vi "VisualizeStatus.vi"() -> ()   [LabVIEW 2014]
uses:
  VisializeBase_class/VisualizeBase_class.lvclass
  <vilib>/Utility/error.llb/Error Cluster From Error Code.vi
  <vilib>/ErrorRing/Error Ring.xnode
  <userlib>/NIST/NISTErrorLib/NISTErrorLib.lvlib
  <vilib>/event_ctls.llb/usereventprio.ctl
  VisializeBase_class/Requests/clUserEventType.ctl
  Framework/Bus_class/Bus_class.lvlib
  Framework/Bus_class/Broadcast/Typedefs/clDidInit.ctl
  Framework/Bus_class/Bus.lvclass
  <vilib>/Utility/miscctls.llb/LVStringsAndValuesArrayTypeDef_U8.ctl
  Events/EventModule/EventModule.lvlib
  PmuImpairment/PmuImpairModule/PmuImpairModule.lvlib
  NetworkImpairment/NetworkImpairmentModule/NetworkImpairmentModule.lvlib
  FlagImpairment/FlagImpairModule/FlagImpairModule.lvlib
  Events/EventPlugins/EventPluginBaseClass/TypeDefs/clEvtReport.ctl
  Events/EventPlugins/EventPluginBaseClass/EventPluginBaseClass.lvclass
  Events/EventPlugins/EventPluginBaseClass/TypeDefs/clEvtReportArray.ctl
  QMH/Typedefs/clEvtRptArray.ctl
  VisializeBase_class/Typedefs/VisualizeData.ctl
  Events/EventPlugins/EventPluginBaseClass/TypeDefs/dblEvtSignalArray.ctl
  QMH/Typedefs/clEvtRptSignal.ctl
  QMH/Typedefs/clPmuImpairRptArray.ctl
  NetworkImpairment/NetworkImpairmentModule/PublicAPI/Arguments/Broadcasts/dblNetworkTime.ctl
  QMH/Typedefs/clNetImpairmentTime.ctl
  NetworkImpairment/NetworkImpairmentModule/PublicAPI/Arguments/Broadcasts/dblPktLoss.ctl
  QMH/Typedefs/clNetIPktLoss.ctl
  FlagImpairment/FlagImpairModule/PublicAPI/Arguments/Broadcasts/ui32FlagImpairmentArray.ctl
  QMH/Typedefs/clFlagImpairArray.ctl
  VisializeBase_class/Typedefs/clVisualizeData.ctl
panel:
  in  "Scrollbar":i32(c297)=20
  in  "QueName":string="FlagQue"
  out "appended array":errorcluster[][](array[cluster])
  in  "btnStop":bool
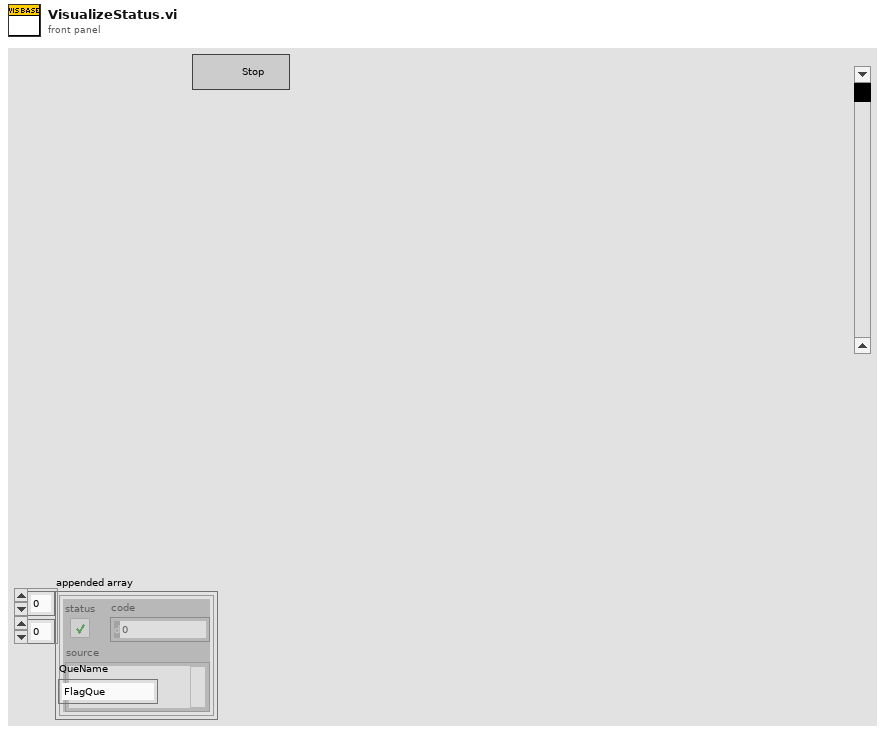
[diagram p1: front panel]
types:
  T1 = typedef "Visualization.lvlib/VisualizeBase_class.lvclass/VisualizeData.ctl" = T2[]
  T2 = typedef "clVisualizeData.ctl" = cluster{"clEvtReportArray":T3, "dblEventSignalArray":T5, "clPmuImpairRptArray":T3, "dblNetworkTime":T6, "dblPktLoss":T7, "FlagImpairArray":T8, "TimeArray":dbl[]}
  T3 = typedef "EventPlugins.lvlib/EventPluginBaseClass.lvclass/clEvtReportArray.ctl" = T4[]
  T4 = typedef "EventPlugins.lvlib/EventPluginBaseClass.lvclass/clEvtReport.ctl" = cluster{"Timestamp":dbl, "Synx":cdb[], "Freq":dbl, "ROCOF":dbl, "ID":i16}
  T5 = typedef "EventPlugins.lvlib/EventPluginBaseClass.lvclass/dblEvtSignalArray.ctl" = dbl[][]
  T6 = typedef "NetworkImpairmentModule.lvlib/dblNetworkTime.ctl" = dbl[]
  T7 = typedef "NetworkImpairmentModule.lvlib/dblPktLoss.ctl" = dbl[]
  T8 = typedef "FlagImpairModule.lvlib/ui32FlagImpairmentArray.ctl" = u32[]
  T9 = typedef "Visualization.lvlib/VisualizeBase_class.lvclass/clRequestEvents.ctl" = cluster{"StopRequest":refnum<user-event>}
  T10 = typedef "Bus_class.lvlib/clBroadcastEvents.ctl" = cluster{"DidInit":refnum<user-event>, "DidStop":refnum<user-event>}
  T11 = typedef "EventModule.lvlib/clBroadcastEvents.ctl" = cluster{"DidInit":refnum<user-event>, "StatusUpdate":refnum<user-event>, "ErrorReport":refnum<user-event>, "DidStop":refnum<user-event>, "ReadEvtConfig":refnum<user-event>, "ReadTimeArray":refnum<user-event>, "ReadEvtParams":refnum<user-event>, "GetEvtReportArray":refnum<user-event>, "ReadPathToPlugin":refnum<user-event>, "GetEvtSignal":refnum<user-event>, "ReadBusNumber":refnum<user-event>}
  T12 = typedef "PmuImpairModule.lvlib/clBroadcastEvents.ctl" = cluster{"DidInit":refnum<user-event>, "StatusUpdate":refnum<user-event>, "ErrorReport":refnum<user-event>, "DidStop":refnum<user-event>, "ImpairConfig":refnum<user-event>, "ImpairParams":refnum<user-event>, "ImpairReports":refnum<user-event>, "PathToPlugin":refnum<user-event>, "BusNumber":refnum<user-event>}
  T13 = typedef "NetworkImpairmentModule.lvlib/clBroadcastEvents.ctl" = cluster{"DidInit":refnum<user-event>, "StatusUpdate":refnum<user-event>, "ErrorReport":refnum<user-event>, "DidStop":refnum<user-event>, "ReadNetImpParams":refnum<user-event>, "ReadLossThreshold":refnum<user-event>, "GetNetworkTime":refnum<user-event>, "GetPktLoss":refnum<user-event>, "ReadPathToPlugin":refnum<user-event>}
  T14 = typedef "FlagImpairModule.lvlib/clBroadcastEvents.ctl" = cluster{"DidInit":refnum<user-event>, "StatusUpdate":refnum<user-event>, "ErrorReport":refnum<user-event>, "DidStop":refnum<user-event>, "ReadFlagImpairConfig":refnum<user-event>, "ReadPluginINIFilePath":refnum<user-event>, "ReadFlagImpairParams":refnum<user-event>, "ReadTimeArray":refnum<user-event>, "GetFlagImpairment":refnum<user-event>}
  T15 = typedef "LVStringsAndValuesArrayTypeDef_U8.ctl" = cluster{"String":string, "Value":u8}[]
  T16 = typedef "Visualization.lvlib/VisualizeBase_class.lvclass/clEvtRptArray.ctl" = cluster{"BusIndex":i32, "clImpairReportArray":T3}
  T17 = typedef "Visualization.lvlib/VisualizeBase_class.lvclass/clPmuImpairRptArray.ctl" = cluster{"BusIndex":i32, "clImpairReportArray":T3}
  T18 = typedef "Visualization.lvlib/VisualizeBase_class.lvclass/clNetImpairmentTime.ctl" = cluster{"BusIndex":i32, "clNetImpairTimeArray":T6}
  T19 = typedef "Visualization.lvlib/VisualizeBase_class.lvclass/clNetIPktLoss.ctl" = cluster{"BusIndex":i32, "clNetPktLoss":T7}
  T20 = typedef "Visualization.lvlib/VisualizeBase_class.lvclass/clFlagImpairArray.ctl" = cluster{"BusIndex":i32, "FlagImpairArray":T8}
  T21 = typedef "Visualization.lvlib/VisualizeBase_class.lvclass/clEvtRptSignal.ctl" = cluster{"BusIndex":i32, "dblEventSignalArray":T5}
  T22 = typedef "Visualization.lvlib/VisualizeBase_class.lvclass/clUserEventType.ctl" = cluster{"BusIndex":i8, "Data":variant}
  T23 = typedef "usereventprio.ctl" = enum32{"high priority", "normal priority"}
  T24 = typedef "Bus_class.lvlib/clDidInit.ctl" = cluster{"Bus":refnum<vi>, "Init?":bool}
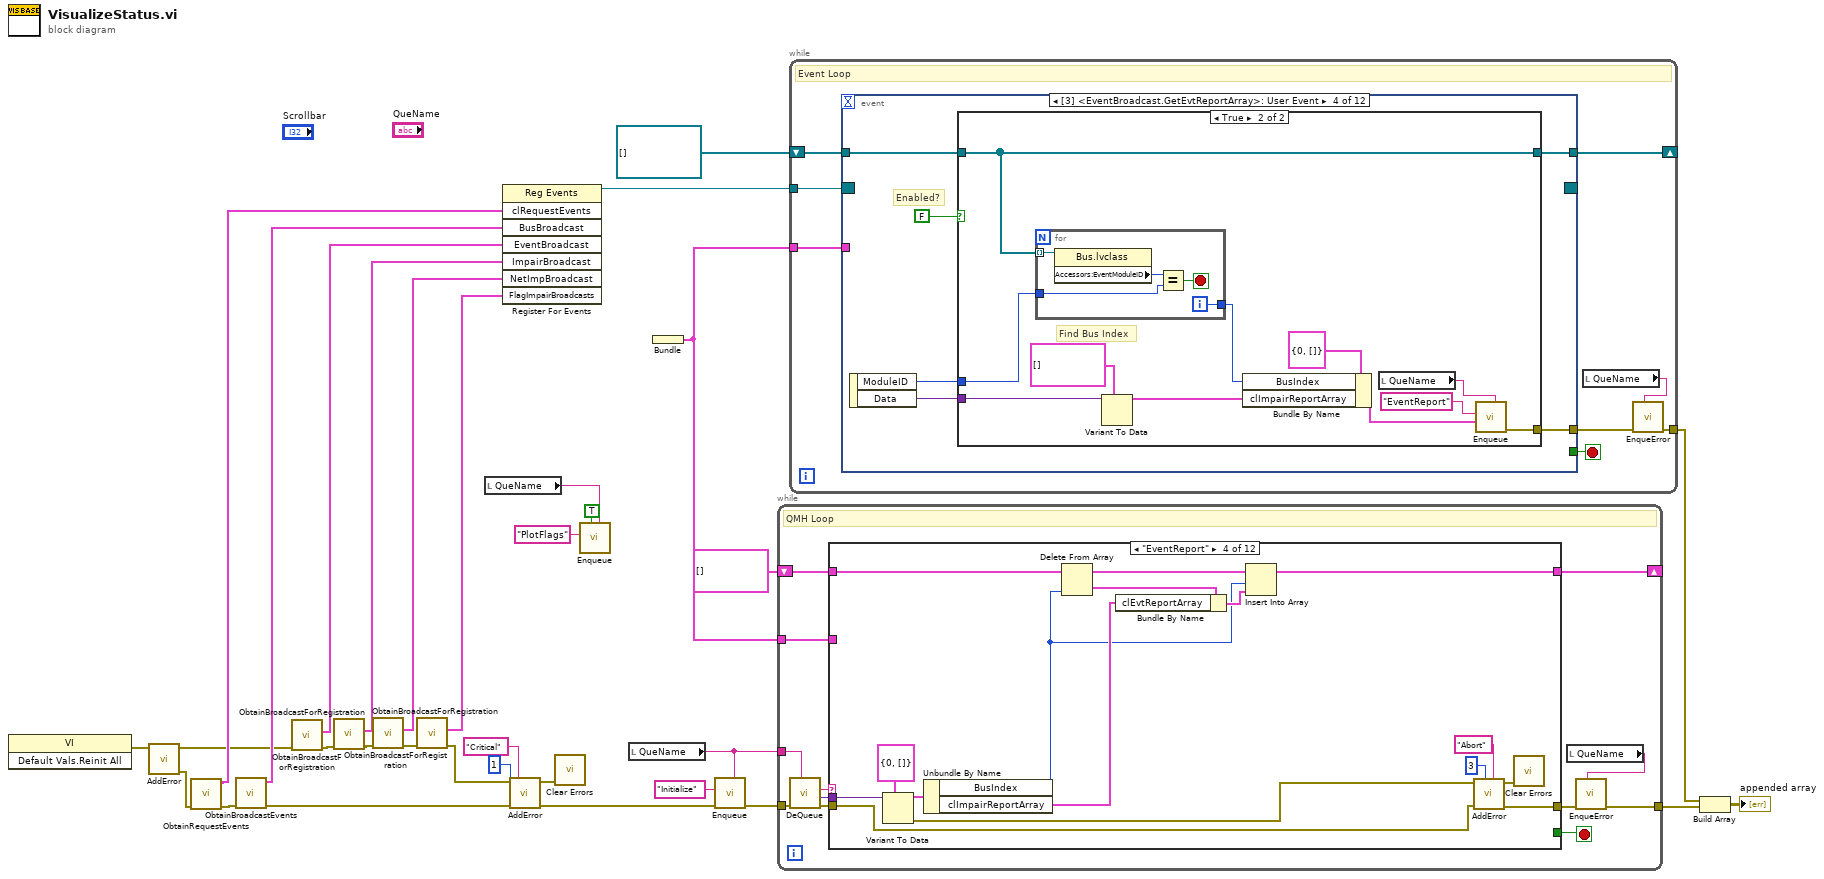
[diagram p0: block diagram]
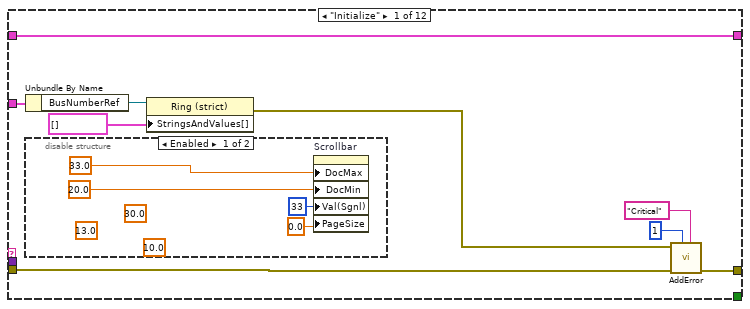
[diagram p2: hidden frame]
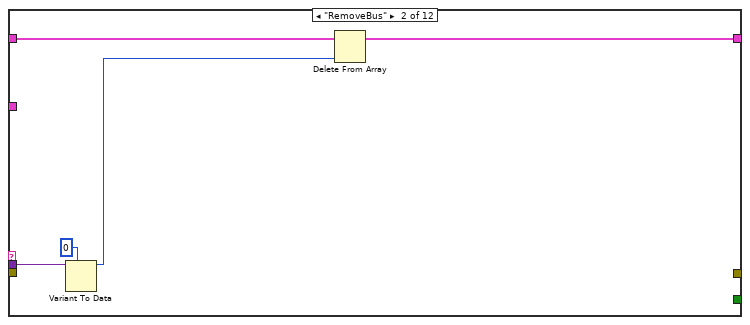
[diagram p4: hidden frame]
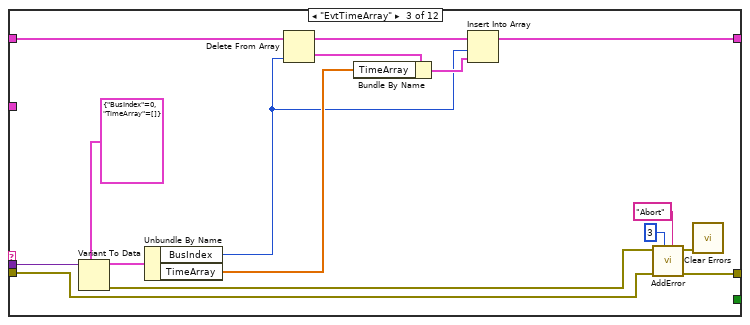
[diagram p5: hidden frame]
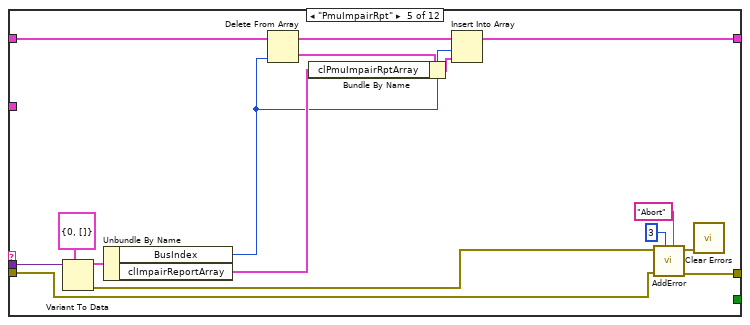
[diagram p6: hidden frame]
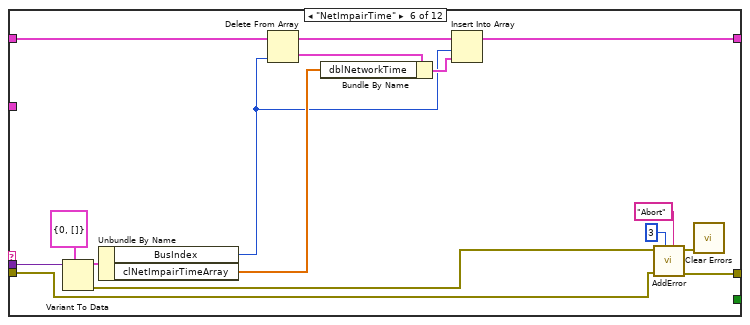
[diagram p7: hidden frame]
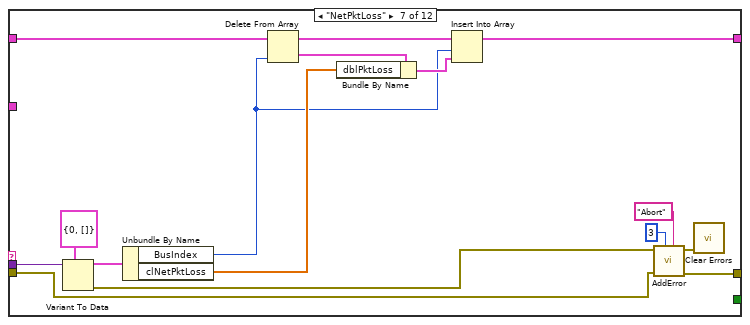
[diagram p8: hidden frame]
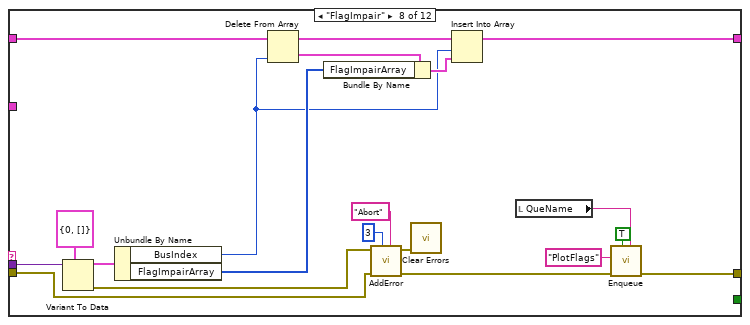
[diagram p9: hidden frame]
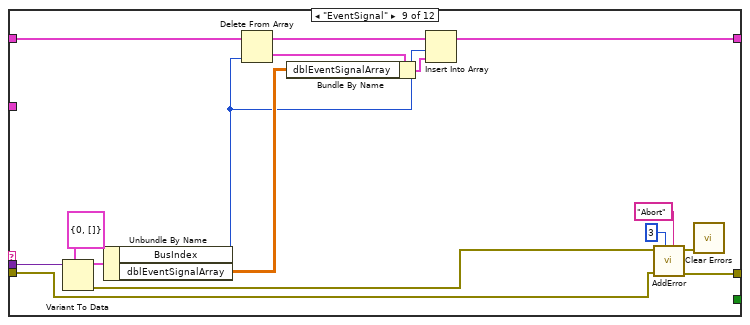
[diagram p10: hidden frame]
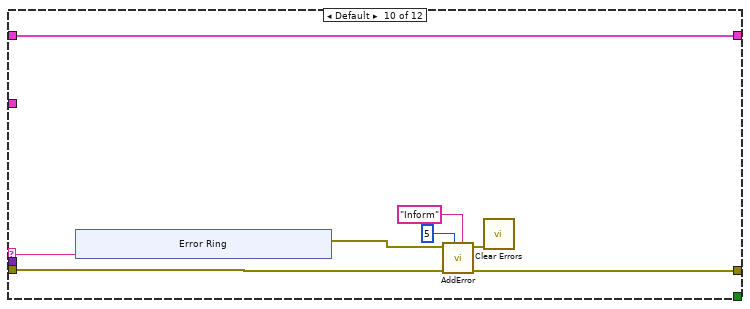
[diagram p11: hidden frame]
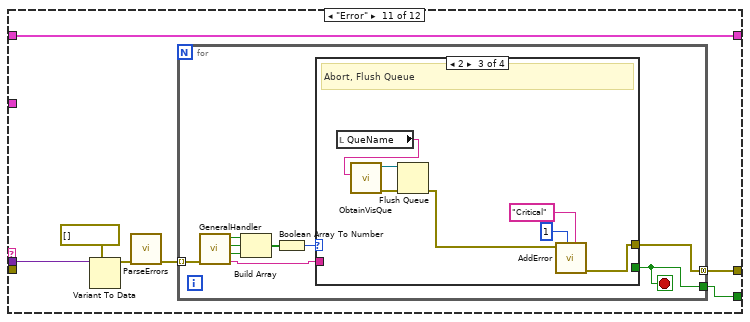
[diagram p12: hidden frame]
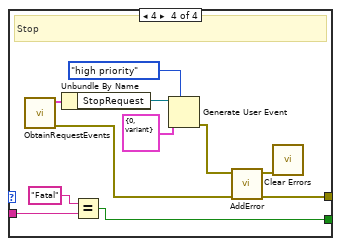
[diagram p15: hidden frame]
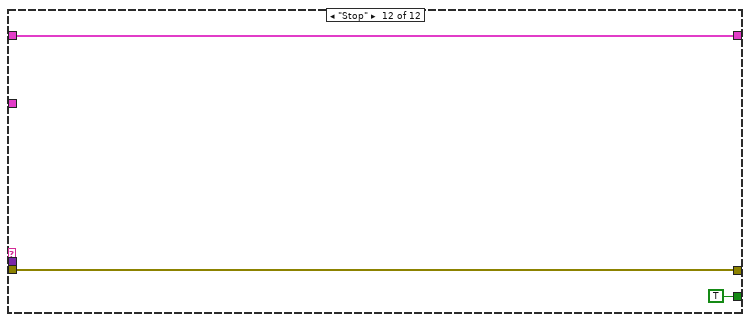
[diagram p16: hidden frame]
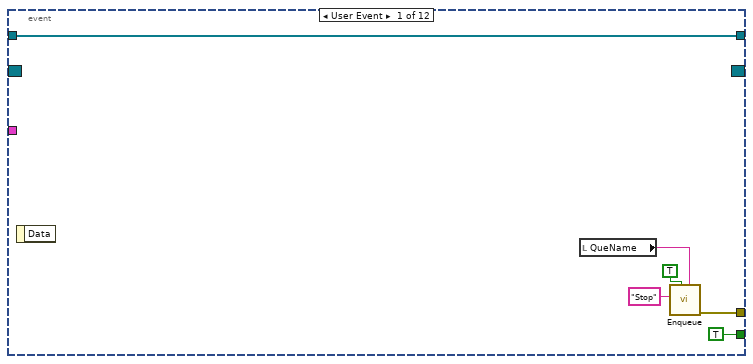
[diagram p17: hidden frame]
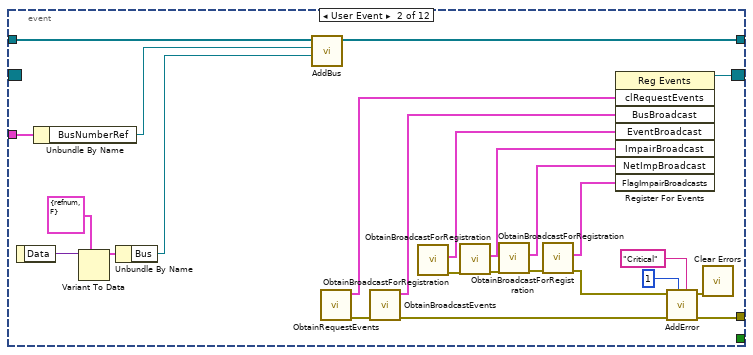
[diagram p18: hidden frame]
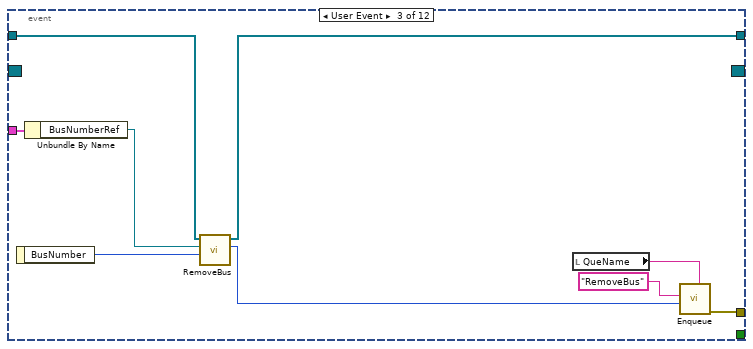
[diagram p19: hidden frame]
diagram:
  n1 = invoke class="VI" method="Default Vals.Reinit All"() -> (error out=w22:errorcluster)  [unwired: 3 in, 2 out]
  n2 = call <userlib>:"AddError.vi"("error in (no error)"=w22) -> ("ErrorArray"=w21:errorcluster[], "error out"=w13:errorcluster)  [unwired: 9 in]
  n3 = call "ObtainRequestEvents.vi"("Error"=w21) -> ("Error"=w26:errorcluster[], "clRequestEvents"=w31:T9)  [unwired: 9 in]
  n4 = call "ObtainBroadcastEvents.vi"("ErrorArray"=w26) -> ("ErrorArray"=w12:errorcluster[], "BusBroadcast"=w25:T10)  [unwired: 9 in]
  n5 = call "ObtainBroadcastForRegistration.vi"("error in (no error)"=w13) -> ("error out"=w16:errorcluster, "EventBroadcast"=w20:T11)  [unwired: 9 in]
  n6 = call "ObtainBroadcastForRegistration.vi"("error in (no error)"=w16) -> ("error out"=w15:errorcluster, "ImpairBroadcast"=w19:T12)  [unwired: 9 in]
  n7 = call "ObtainBroadcastForRegistration.vi"("error in (no error)"=w15) -> ("error out"=w14:errorcluster, "NetImpBroadcast"=w18:T13)  [unwired: 9 in]
  n8 = call "ObtainBroadcastForRegistration.vi"("error in (no error)"=w14) -> ("error out"=w11:errorcluster, "FlagImpairBroadcasts"=w17:T14)  [unwired: 9 in]
  n9 = local read "QueName"() -> (w3:string)
  n10 = register-events(w31, w25, w20, w19, w18, w17) -> (reference out=w30:refnum<event-registration>)  [unwired: 2 in, 1 out]
  n11 = call <userlib>:"AddError.vi"("Severity"="Critical" ("String"), "Priority"=u8 1, "ErrorArray"=w12, "error in (no error)"=w11) -> ("ErrorArray"=w8:errorcluster[], "error out"=w5:errorcluster)  [unwired: 6 in]
  n12 = call <vilib>:"Clear Errors.vi"("error in (no error)"=w5) -> ()  [unwired: 5 in, 2 out]
  n13 = call "Enqueue.vi"("QueName"=w3, "Priority? (F)"=TRUE, "Message"="PlotFlags") -> ()  [unwired: 8 in, 1 out]
  n14 = local read "QueName"() -> (w4:string)
  n15 = Bundle() -> (w6:cluster{void}, w24)  [unwired: 1 in]
  n16 = call "Enqueue.vi"("QueName"=w4, "Error"=w8, "Message"="Initialize") -> ("Error"=w32:errorcluster[])  [unwired: 8 in]
  n17 = while {
    tunnel: w32 -> [w45]
    tunnel: [w39] -> w29
    tunnel: w6 -> [w38]
    shift-right: [w36] -> _
    shift-left: T1 [] ("VisualizeData") -> [w37]
    tunnel: w4 -> [w35]
    stop <- w40 stop-if-true
    # "QMH Loop"
    n18 = call "DeQueue.vi"("QueName"=w35, "Error"=w45) -> ("Error"=w42:errorcluster[], "Data"=w43:variant, "Message"=w44:string)  [unwired: 7 in]
    n19 = case shown="\"EventReport\"" w44 {
      selector: w44 -> [_ _ _ _ _ _ _ _ _ w190 _ _]
      tunnel: w43 -> [_ w66 w69 w98 w114 w130 w146 w166 w182 _ w204 _]
      tunnel: w42 -> [w51 _ w68 w83 w99 w115 w131 w152 w167 w188 _ w233]
      tunnel: [w50 _ w67 w88 w104 w120 w136 w150 w172 w187 w200 w233] -> w41
      tunnel: [_ _ _ _ _ _ _ _ _ _ w199 TRUE] -> w40
      tunnel: w38 -> [w54 _ _ _ _ _ _ _ _ _ _ _]
      tunnel: w37 -> [w46 w64 w71 w94 w110 w126 w142 w162 w178 w183 w198 w232]
      tunnel: [w46 w63 w70 w95 w111 w127 w143 w163 w179 w183 w198 w232] -> w36
      frame "Initialize" {
        n20 = Unbundle By Name(w54) -> ("BusNumberRef"=w53:refnum<vi>)
        n21 = disable-structure shown="Enabled" {
          frame Enabled {
            w55 = 10.0 ("Y Scale.Range:Increment")
            w59 = 30.0 ("Y Scale.Range:Maximum")
            w58 = 13.0 ("Y Scale.Range:Maximum")
            n22 = property on="Scrollbar" class="Scroll (strict)"("DocMax"=33.0 ("Doc Max"), "DocMin"=20.0 ("Doc Min"), "Val(Sgnl)"=33 ("Scrollbar"), "PageSize"=0.0 ("Page Size")) -> ()  [unwired: 2 in, 2 out]
          }
          frame Disabled {
          }
        }
        n23 = property class="Ring (strict)"(reference=w53, "StringsAndValues[]"=T15 [] ("Strings And Values []")) -> (error out=w49:errorcluster)  [unwired: 1 in, 1 out]
        n24 = call <userlib>:"AddError.vi"("Severity"="Critical" ("String"), "Priority"=u8 1, "ErrorArray"=w51, "error in (no error)"=w49) -> ("ErrorArray"=w50:errorcluster[])  [unwired: 6 in, 1 out]
      }
      frame "RemoveBus" {
        n25 = Variant To Data(type=0, Variant=w66) -> (data=w62:i32)  [unwired: 1 in, 1 out]
        n26 = Delete From Array(array=w64, index=w62) -> (array with subset deleted=w63:T1)  [unwired: 1 in, 1 out]
      }
      frame "EvtTimeArray" {
        n27 = Variant To Data(type=cluster{"BusIndex":i32, "TimeArray":dbl[]} {"BusIndex"=0, "TimeArray"=[]} ("cluster"), Variant=w69) -> (data=w78:cluster{"BusIndex":i32, "TimeArray":dbl[]}, error out=w82:errorcluster)  [unwired: 1 in]
        n28 = Unbundle By Name(w78) -> ("BusIndex"=w73:i32, "TimeArray"=w75:dbl[])
        n29 = Delete From Array(array=w71, index=w73) -> (deleted portion=w76:T2, array with subset deleted=w77:T1)  [unwired: 1 in]
        n30 = Bundle By Name(cluster=w76, "TimeArray"=w75) -> (w74:T2)
        n31 = Insert Into Array(array=w77, index=w73, new element=w74) -> (w70:T1)
        n32 = call <userlib>:"AddError.vi"("Severity"="Abort" ("String"), "Priority"=u8 3, "ErrorArray"=w68, "error in (no error)"=w82) -> ("ErrorArray"=w67:errorcluster[], "error out"=w81:errorcluster)  [unwired: 6 in]
        n33 = call <vilib>:"Clear Errors.vi"("error in (no error)"=w81) -> ()  [unwired: 5 in, 2 out]
      }
      frame "EventReport" {
        n34 = Variant To Data(type=T16 {"BusIndex"=0, "clImpairReportArray"=[]} ("clEvtReportArray"), Variant=w98) -> (data=w96:T16, error out=w87:errorcluster)  [unwired: 1 in]
        n35 = Unbundle By Name(w96) -> ("BusIndex"=w89:i32, "clImpairReportArray"=w91:T3)
        n36 = Delete From Array(array=w94, index=w89) -> (deleted portion=w92:T2, array with subset deleted=w93:T1)  [unwired: 1 in]
        n37 = Bundle By Name(cluster=w92, "clEvtReportArray"=w91) -> (w90:T2)
        n38 = Insert Into Array(array=w93, index=w89, new element=w90) -> (w95:T1)
        n39 = call <userlib>:"AddError.vi"("Severity"="Abort" ("String"), "Priority"=u8 3, "ErrorArray"=w83, "error in (no error)"=w87) -> ("ErrorArray"=w88:errorcluster[], "error out"=w86:errorcluster)  [unwired: 6 in]
        n40 = call <vilib>:"Clear Errors.vi"("error in (no error)"=w86) -> ()  [unwired: 5 in, 2 out]
      }
      frame "PmuImpairRpt" {
        n41 = Variant To Data(type=T17 {"BusIndex"=0, "clImpairReportArray"=[]} ("clImpairReportArray"), Variant=w114) -> (data=w112:T17, error out=w103:errorcluster)  [unwired: 1 in]
        n42 = Unbundle By Name(w112) -> ("BusIndex"=w105:i32, "clImpairReportArray"=w107:T3)
        n43 = Delete From Array(array=w110, index=w105) -> (deleted portion=w108:T2, array with subset deleted=w109:T1)  [unwired: 1 in]
        n44 = Bundle By Name(cluster=w108, "clPmuImpairRptArray"=w107) -> (w106:T2)
        n45 = Insert Into Array(array=w109, index=w105, new element=w106) -> (w111:T1)
        n46 = call <userlib>:"AddError.vi"("Severity"="Abort" ("String"), "Priority"=u8 3, "ErrorArray"=w99, "error in (no error)"=w103) -> ("ErrorArray"=w104:errorcluster[], "error out"=w102:errorcluster)  [unwired: 6 in]
        n47 = call <vilib>:"Clear Errors.vi"("error in (no error)"=w102) -> ()  [unwired: 5 in, 2 out]
      }
      frame "NetImpairTime" {
        n48 = Variant To Data(type=T18 {"BusIndex"=0, "clNetImpairTimeArray"=[]} ("clImpairReportArray"), Variant=w130) -> (data=w128:T18, error out=w119:errorcluster)  [unwired: 1 in]
        n49 = Unbundle By Name(w128) -> ("BusIndex"=w121:i32, "clNetImpairTimeArray"=w123:T6)
        n50 = Delete From Array(array=w126, index=w121) -> (deleted portion=w124:T2, array with subset deleted=w125:T1)  [unwired: 1 in]
        n51 = Bundle By Name(cluster=w124, "dblNetworkTime"=w123) -> (w122:T2)
        n52 = Insert Into Array(array=w125, index=w121, new element=w122) -> (w127:T1)
        n53 = call <userlib>:"AddError.vi"("Severity"="Abort" ("String"), "Priority"=u8 3, "ErrorArray"=w115, "error in (no error)"=w119) -> ("ErrorArray"=w120:errorcluster[], "error out"=w118:errorcluster)  [unwired: 6 in]
        n54 = call <vilib>:"Clear Errors.vi"("error in (no error)"=w118) -> ()  [unwired: 5 in, 2 out]
      }
      frame "NetPktLoss" {
        n55 = Variant To Data(type=T19 {"BusIndex"=0, "clNetPktLoss"=[]} ("clNetPktLoss"), Variant=w146) -> (data=w144:T19, error out=w135:errorcluster)  [unwired: 1 in]
        n56 = Unbundle By Name(w144) -> ("BusIndex"=w137:i32, "clNetPktLoss"=w139:T7)
        n57 = Delete From Array(array=w142, index=w137) -> (deleted portion=w140:T2, array with subset deleted=w141:T1)  [unwired: 1 in]
        n58 = Bundle By Name(cluster=w140, "dblPktLoss"=w139) -> (w138:T2)
        n59 = Insert Into Array(array=w141, index=w137, new element=w138) -> (w143:T1)
        n60 = call <userlib>:"AddError.vi"("Severity"="Abort" ("String"), "Priority"=u8 3, "ErrorArray"=w131, "error in (no error)"=w135) -> ("ErrorArray"=w136:errorcluster[], "error out"=w134:errorcluster)  [unwired: 6 in]
        n61 = call <vilib>:"Clear Errors.vi"("error in (no error)"=w134) -> ()  [unwired: 5 in, 2 out]
      }
      frame "FlagImpair" {
        n62 = Variant To Data(type=T20 {"BusIndex"=0, "FlagImpairArray"=[]} ("clFlagImpairArray"), Variant=w166) -> (data=w164:T20, error out=w156:errorcluster)  [unwired: 1 in]
        n63 = Unbundle By Name(w164) -> ("BusIndex"=w157:i32, "FlagImpairArray"=w159:T8)
        n64 = Delete From Array(array=w162, index=w157) -> (deleted portion=w160:T2, array with subset deleted=w161:T1)  [unwired: 1 in]
        n65 = Bundle By Name(cluster=w160, "FlagImpairArray"=w159) -> (w158:T2)
        n66 = call <userlib>:"AddError.vi"("Severity"="Abort" ("String"), "Priority"=u8 3, "ErrorArray"=w152, "error in (no error)"=w156) -> ("ErrorArray"=w151:errorcluster[], "error out"=w155:errorcluster)  [unwired: 6 in]
        n67 = call <vilib>:"Clear Errors.vi"("error in (no error)"=w155) -> ()  [unwired: 5 in, 2 out]
        n68 = Insert Into Array(array=w161, index=w157, new element=w158) -> (w163:T1)
        n69 = local read "QueName"() -> (w147:string)
        n70 = call "Enqueue.vi"("QueName"=w147, "Priority? (F)"=TRUE, "Error"=w151, "Message"="PlotFlags") -> ("Error"=w150:errorcluster[])  [unwired: 7 in]
      }
      frame "EventSignal" {
        n71 = Variant To Data(type=T21 {"BusIndex"=0, "dblEventSignalArray"=[]} ("clEvtReportArray"), Variant=w182) -> (data=w180:T21, error out=w171:errorcluster)  [unwired: 1 in]
        n72 = Unbundle By Name(w180) -> ("BusIndex"=w173:i32, "dblEventSignalArray"=w175:T5)
        n73 = Delete From Array(array=w178, index=w173) -> (deleted portion=w176:T2, array with subset deleted=w177:T1)  [unwired: 1 in]
        n74 = Bundle By Name(cluster=w176, "dblEventSignalArray"=w175) -> (w174:T2)
        n75 = Insert Into Array(array=w177, index=w173, new element=w174) -> (w179:T1)
        n76 = call <userlib>:"AddError.vi"("Severity"="Abort" ("String"), "Priority"=u8 3, "ErrorArray"=w167, "error in (no error)"=w171) -> ("ErrorArray"=w172:errorcluster[], "error out"=w170:errorcluster)  [unwired: 6 in]
        n77 = call <vilib>:"Clear Errors.vi"("error in (no error)"=w170) -> ()  [unwired: 5 in, 2 out]
      }
      frame Default {
        n78 = xnode "Error Ring"("parameter 0"=w190) -> ("error out"=w189:errorcluster)
        n79 = call <userlib>:"AddError.vi"("Severity"="Inform" ("String"), "Priority"=u8 5, "ErrorArray"=w188, "error in (no error)"=w189) -> ("ErrorArray"=w187:errorcluster[], "error out"=w186:errorcluster)  [unwired: 6 in]
        n80 = call <vilib>:"Clear Errors.vi"("error in (no error)"=w186) -> ()  [unwired: 5 in, 2 out]
      }
      frame "Error" {
        n81 = Variant To Data(type=errorcluster[] [], Variant=w204) -> (data=w202:errorcluster[])  [unwired: 1 in, 1 out]
        n82 = call <userlib>:"ParseErrors.vi"("ErrorArray"=w202) -> ("ErrorArray"=w201:errorcluster[])  [unwired: 8 in, 2 out]
        n83 = for {
          tunnel: w201 -> [w213] mode=indexing
          tunnel: [w207] -> w200 mode=concatenating
          tunnel: [w205] -> w199
          stop <- w205 stop-if-true
          n84 = call <userlib>:"GeneralHandler.vi"("error in (no error)"=w213) -> ("Severity"=w206:string, "Stop"=w210:bool, "Abort"=w211:bool, "Continue"=w212:bool)  [unwired: 7 in]
          n85 = Build Array(w212, w211, w210) -> (w209:bool[])
          n86 = Boolean Array To Number(Boolean array=w209) -> (number=w208:u32)
          n87 = case shown="2" w208 {
            tunnel: [_ _ w218 w229] -> w207
            tunnel: w206 -> [_ _ _ w223]
            tunnel: [_ _ _ w221] -> w205
            frame 0, Default {
              # "No Dialog"
            }
            frame 1 {
              # "Continue"
            }
            frame 2 {
              # "Abort, Flush Queue"
              n88 = local read "QueName"() -> (w214:string)
              n89 = call "ObtainVisQue.vi"("QueName"=w214) -> ("error out"=w220:errorcluster, "queue out"=w219:refnum<queue>)  [unwired: 9 in]
              n90 = Flush Queue(queue=w219, error in (no error)=w220) -> (error out=w217:errorcluster)  [unwired: 2 out]
              n91 = call <userlib>:"AddError.vi"("Severity"="Critical" ("String"), "Priority"=u8 1, "error in (no error)"=w217) -> ("ErrorArray"=w218:errorcluster[])  [unwired: 7 in, 1 out]
            }
            frame 4 {
              # "Stop"
              n92 = call "ObtainRequestEvents.vi"() -> ("Error"=w227:errorcluster[], "clRequestEvents"=w231:T9)  [unwired: 10 in]
              n93 = Unbundle By Name(w231) -> ("StopRequest"=w230:refnum<user-event>)
              n94 = Equal?(x="Fatal", y=w223) -> (x = y?=w221:bool)
              n95 = Generate User Event(priority (normal)=usereventprio."high priority", user event=w230, event data cluster=T22 {"BusIndex"=0, "Data"=variant} ("event data")) -> (error out=w228:errorcluster)  [unwired: 1 in, 1 out]
              n96 = call <userlib>:"AddError.vi"("ErrorArray"=w227, "error in (no error)"=w228) -> ("ErrorArray"=w229:errorcluster[], "error out"=w224:errorcluster)  [unwired: 8 in]
              n97 = call <vilib>:"Clear Errors.vi"("error in (no error)"=w224) -> ()  [unwired: 5 in, 2 out]
            }
          }
        }
      }
      frame "Stop" {
      }
    }
    n98 = local read "QueName"() -> (w34:string)
    n99 = call "EnqueError.vi"("QueName"=w34, "Error"=w41) -> ("Error"=w39:errorcluster[])  [unwired: 9 in]
  }
  n100 = while {
    tunnel: w30 -> [w242]
    tunnel: [w239] -> w28
    tunnel: w6 -> [w238]
    shift-right: [w236] -> _
    shift-left: refnum<class "Bus.lvclass">[] [] -> [w237]
    stop <- w241 stop-if-true
    # "Event Loop"
    n101 = event shown="[3] <EventBroadcast.GetEvtReportArray>: User Event" {
      selector: w242 -> [_ _ _ _ _ _ _ _ _ _ _ _]
      dyn-events: [_ w257 _ _ _ _ _ _ _ _ _ _] -> _
      timeout: _ -> [_ _ _ _ _ _ _ _ _ _ _ _]
      tunnel: [TRUE _ _ _ _ _ _ _ _ _ _ _] -> w241
      tunnel: [w247 w260 w278 w285 w311 w336 w359 w382 w405 w428 _ w461] -> w240
      tunnel: w238 -> [_ w270 w282 _ _ _ _ _ _ _ _ _]
      tunnel: w237 -> [w244 w269 w281 w288 w309 w339 w362 w385 w408 w431 w449 w455]
      tunnel: [w244 w266 w280 w283 w310 w334 w357 w380 w403 w426 w449 w455] -> w236
      event User Event {
        n102 = event-data() -> ()  [unwired: 1 in, 1 out]
        n103 = local read "QueName"() -> (w243:string)
        n104 = call "Enqueue.vi"("QueName"=w243, "Priority? (F)"=TRUE, "Message"="Stop") -> ("Error"=w247:errorcluster[])  [unwired: 8 in]
      }
      event User Event {
        n105 = event-data() -> ("Data"=w273:variant)  [unwired: 1 in]
        n106 = Unbundle By Name(w270) -> ("BusNumberRef"=w268:refnum<vi>)
        n107 = Variant To Data(type=T24 {"Bus"=refnum, "Init?"=FALSE} ("clBusDidInit"), Variant=w273) -> (data=w271:T24)  [unwired: 1 in, 1 out]
        n108 = Unbundle By Name(w271) -> ("Bus"=w267:refnum<vi>)
        n109 = call "AddBus.vi"("BusRef"=w267, "BusNumberRef"=w268, "BusArray"=w269) -> ("BusArray"=w266:refnum<class "Bus.lvclass">[])  [unwired: 8 in]
        n110 = call "ObtainRequestEvents.vi"() -> ("Error"=w252:errorcluster[], "clRequestEvents"=w250:T9)  [unwired: 10 in]
        n111 = call "ObtainBroadcastEvents.vi"("ErrorArray"=w252) -> ("ErrorArray"=w251:errorcluster[], "BusBroadcast"=w249:T10)  [unwired: 9 in]
        n112 = call "ObtainBroadcastForRegistration.vi"() -> ("error out"=w265:errorcluster, "EventBroadcast"=w256:T11)  [unwired: 10 in]
        n113 = call "ObtainBroadcastForRegistration.vi"("error in (no error)"=w265) -> ("error out"=w264:errorcluster, "ImpairBroadcast"=w255:T12)  [unwired: 9 in]
        n114 = call "ObtainBroadcastForRegistration.vi"("error in (no error)"=w264) -> ("error out"=w263:errorcluster, "NetImpBroadcast"=w254:T13)  [unwired: 9 in]
        n115 = call "ObtainBroadcastForRegistration.vi"("error in (no error)"=w263) -> ("error out"=w258:errorcluster, "FlagImpairBroadcasts"=w253:T14)  [unwired: 9 in]
        n116 = register-events(w250, w249, w256, w255, w254, w253) -> (reference out=w257:refnum<event-registration>)  [unwired: 2 in, 1 out]
        n117 = call <userlib>:"AddError.vi"("Severity"="Critical" ("String"), "Priority"=u8 1, "ErrorArray"=w251, "error in (no error)"=w258) -> ("ErrorArray"=w260:errorcluster[], "error out"=w259:errorcluster)  [unwired: 6 in]
        n118 = call <vilib>:"Clear Errors.vi"("error in (no error)"=w259) -> ()  [unwired: 5 in, 2 out]
      }
      event User Event {
        n119 = event-data() -> ("BusNumber"=w275:i8)  [unwired: 1 in]
        n120 = Unbundle By Name(w282) -> ("BusNumberRef"=w279:refnum<vi>)
        n121 = call "RemoveBus.vi"("BusArray"=w281, "BusNumberRef"=w279, "BusNumber"=w275) -> ("BusArray"=w280:refnum<class "Bus.lvclass">[], "BusIndex"=w277:i32)  [unwired: 6 in]
        n122 = local read "QueName"() -> (w274:string)
        n123 = call "Enqueue.vi"("QueName"=w274, "Data"=w277, "Message"="RemoveBus") -> ("Error"=w278:errorcluster[])  [unwired: 8 in]
      }
      event User Event {
        # "Enabled?"
        n124 = event-data() -> ("ModuleID"=w287:i32, "Data"=w286:variant)  [unwired: 1 in]
        n125 = case shown="True" FALSE {
          tunnel: w288 -> [w289 w291]
          tunnel: w287 -> [_ w300]
          tunnel: w286 -> [_ w298]
          tunnel: [_ w295] -> w285
          tunnel: [w289 w291] -> w283
          frame False {
          }
          frame True {
            # "Find Bus Index"
            n126 = for {
              tunnel: w291 -> [w305] mode=indexing
              tunnel: w300 -> [w303]
              tunnel: [w301] -> w299
              i -> [w301]
              stop <- w302 stop-if-true
              n127 = property class="Bus.lvclass"(reference=w305) -> ("Accessors:EventModuleID"=w304:i32)  [unwired: 1 in, 2 out]
              n128 = Equal?(x=w304, y=w303) -> (x = y?=w302:bool)
            }
            n129 = Variant To Data(type=T3 [] ("clEvtReportArray"), Variant=w298) -> (data=w296:T3)  [unwired: 1 in, 1 out]
            n130 = Bundle By Name(cluster=T16 {"BusIndex"=0, "clImpairReportArray"=[]} ("clEvtReportArray"), "BusIndex"=w299, "clImpairReportArray"=w296) -> (w294:T16)
            n131 = local read "QueName"() -> (w290:string)
            n132 = call "Enqueue.vi"("QueName"=w290, "Data"=w294, "Message"="EventReport") -> ("Error"=w295:errorcluster[])  [unwired: 8 in]
          }
        }
      }
      event User Event {
        w306 = TRUE  # Enabled?
        n133 = event-data() -> ("ModuleID"=w308:i32, "Data"=w307:variant)  [unwired: 1 in]
        n134 = case shown="True" w306 {
          tunnel: [w312 w328] -> w310
          tunnel: w309 -> [w312 w328]
          tunnel: w308 -> [_ w325]
          tunnel: w307 -> [_ w327]
          tunnel: [_ w315] -> w311
          frame False {
          }
          frame True {
            n135 = Variant To Data(type=dbl[] [], Variant=w327) -> (data=w324:dbl[], error out=w320:errorcluster)  [unwired: 1 in]
            n136 = for {
              tunnel: w328 -> [w333] mode=indexing
              tunnel: w325 -> [w331]
              tunnel: [w329] -> w314
              i -> [w329]
              stop <- w330 stop-if-true
              # "Find Bus Index"
              n137 = property class="Bus.lvclass"(reference=w333) -> ("Accessors:EventModuleID"=w332:i32)  [unwired: 1 in, 2 out]
              n138 = Equal?(x=w332, y=w331) -> (x = y?=w330:bool)
            }
            n139 = call <userlib>:"AddError.vi"("Severity"="Critical" ("String"), "Priority"=u8 1, "error in (no error)"=w320) -> ("ErrorArray"=w316:errorcluster[], "error out"=w319:errorcluster)  [unwired: 7 in]
            n140 = call <vilib>:"Clear Errors.vi"("error in (no error)"=w319) -> ()  [unwired: 5 in, 2 out]
            n141 = Bundle(w314, w324) -> (w323:cluster{i32, dbl[]})  [unwired: 1 in]
            n142 = To Variant(anything=w323) -> (Variant=w322:variant)
            n143 = local read "QueName"() -> (w313:string)
            n144 = call "Enqueue.vi"("QueName"=w313, "Error"=w316, "Data"=w322, "Message"="EvtTimeArray") -> ("Error"=w315:errorcluster[])  [unwired: 7 in]
          }
        }
      }
      event User Event {
        # "Enabled?"
        n145 = event-data() -> ("ModuleID"=w338:i32, "Data"=w337:variant)  [unwired: 1 in]
        n146 = case shown="False" FALSE {
          tunnel: w339 -> [w340 w342]
          tunnel: w338 -> [_ w351]
          tunnel: w337 -> [_ w349]
          tunnel: [_ w346] -> w336
          tunnel: [w340 w342] -> w334
          frame False {
          }
          frame True {
            # "Find Bus Index"
            n147 = for {
              tunnel: w342 -> [w356] mode=indexing
              tunnel: w351 -> [w354]
              tunnel: [w352] -> w350
              i -> [w352]
              stop <- w353 stop-if-true
              n148 = property class="Bus.lvclass"(reference=w356) -> ("Accessors:EventModuleID"=w355:i32)  [unwired: 1 in, 2 out]
              n149 = Equal?(x=w355, y=w354) -> (x = y?=w353:bool)
            }
            n150 = Variant To Data(type=T5 [] ("dblEventSignalArray"), Variant=w349) -> (data=w347:T5)  [unwired: 1 in, 1 out]
            n151 = Bundle By Name(cluster=T21 {"BusIndex"=0, "dblEventSignalArray"=[]} ("clEvtReportArray"), "BusIndex"=w350, "dblEventSignalArray"=w347) -> (w345:T21)
            n152 = local read "QueName"() -> (w341:string)
            n153 = call "Enqueue.vi"("QueName"=w341, "Data"=w345, "Message"="EventSignal") -> ("Error"=w346:errorcluster[])  [unwired: 8 in]
          }
        }
      }
      event User Event {
        # "Enabled?"
        n154 = event-data() -> ("ModuleID"=w361:i32, "Data"=w360:variant)  [unwired: 1 in]
        n155 = case shown="True" FALSE {
          tunnel: w362 -> [w363 w365]
          tunnel: w361 -> [_ w374]
          tunnel: w360 -> [_ w372]
          tunnel: [_ w369] -> w359
          tunnel: [w363 w365] -> w357
          frame False {
          }
          frame True {
            # "Find Bus Index"
            n156 = for {
              tunnel: w365 -> [w379] mode=indexing
              tunnel: w374 -> [w377]
              tunnel: [w375] -> w373
              i -> [w375]
              stop <- w376 stop-if-true
              n157 = property class="Bus.lvclass"(reference=w379) -> ("Accessors:EventModuleID"=w378:i32)  [unwired: 1 in, 2 out]
              n158 = Equal?(x=w378, y=w377) -> (x = y?=w376:bool)
            }
            n159 = Variant To Data(type=T3 [] ("clEvtReportArray"), Variant=w372) -> (data=w370:T3)  [unwired: 1 in, 1 out]
            n160 = Bundle By Name(cluster=T17 {"BusIndex"=0, "clImpairReportArray"=[]} ("clEvtReportArray"), "BusIndex"=w373, "clImpairReportArray"=w370) -> (w368:T17)
            n161 = local read "QueName"() -> (w364:string)
            n162 = call "Enqueue.vi"("QueName"=w364, "Data"=w368, "Message"="PmuImpairRpt") -> ("Error"=w369:errorcluster[])  [unwired: 8 in]
          }
        }
      }
      event User Event {
        # "Enabled?"
        n163 = event-data() -> ("ModuleID"=w384:i32, "Data"=w383:variant)  [unwired: 1 in]
        n164 = case shown="False" FALSE {
          tunnel: w385 -> [w386 w388]
          tunnel: w384 -> [_ w397]
          tunnel: w383 -> [_ w395]
          tunnel: [_ w392] -> w382
          tunnel: [w386 w388] -> w380
          frame False {
          }
          frame True {
            # "Find Bus Index"
            n165 = for {
              tunnel: w388 -> [w402] mode=indexing
              tunnel: w397 -> [w400]
              tunnel: [w398] -> w396
              i -> [w398]
              stop <- w399 stop-if-true
              n166 = property class="Bus.lvclass"(reference=w402) -> ("Accessors:EventModuleID"=w401:i32)  [unwired: 1 in, 2 out]
              n167 = Equal?(x=w401, y=w400) -> (x = y?=w399:bool)
            }
            n168 = Variant To Data(type=T6 [] ("dblNetworkTime"), Variant=w395) -> (data=w393:T6)  [unwired: 1 in, 1 out]
            n169 = Bundle By Name(cluster=T18 {"BusIndex"=0, "clNetImpairTimeArray"=[]} ("clEvtReportArray"), "BusIndex"=w396, "clNetImpairTimeArray"=w393) -> (w391:T18)
            n170 = local read "QueName"() -> (w387:string)
            n171 = call "Enqueue.vi"("QueName"=w387, "Data"=w391, "Message"="NetImpairTime") -> ("Error"=w392:errorcluster[])  [unwired: 8 in]
          }
        }
      }
      event User Event {
        # "Enabled?"
        n172 = event-data() -> ("ModuleID"=w407:i32, "Data"=w406:variant)  [unwired: 1 in]
        n173 = case shown="False" FALSE {
          tunnel: w408 -> [w409 w411]
          tunnel: w407 -> [_ w420]
          tunnel: w406 -> [_ w418]
          tunnel: [_ w415] -> w405
          tunnel: [w409 w411] -> w403
          frame False {
          }
          frame True {
            # "Find Bus Index"
            n174 = for {
              tunnel: w411 -> [w425] mode=indexing
              tunnel: w420 -> [w423]
              tunnel: [w421] -> w419
              i -> [w421]
              stop <- w422 stop-if-true
              n175 = property class="Bus.lvclass"(reference=w425) -> ("Accessors:EventModuleID"=w424:i32)  [unwired: 1 in, 2 out]
              n176 = Equal?(x=w424, y=w423) -> (x = y?=w422:bool)
            }
            n177 = Variant To Data(type=T7 [] ("dblPktLoss"), Variant=w418) -> (data=w416:T7)  [unwired: 1 in, 1 out]
            n178 = Bundle By Name(cluster=T19 {"BusIndex"=0, "clNetPktLoss"=[]} ("clEvtReportArray"), "BusIndex"=w419, "clNetPktLoss"=w416) -> (w414:T19)
            n179 = local read "QueName"() -> (w410:string)
            n180 = call "Enqueue.vi"("QueName"=w410, "Data"=w414, "Message"="NetPktLoss") -> ("Error"=w415:errorcluster[])  [unwired: 8 in]
          }
        }
      }
      event User Event {
        # "Enabled?"
        n181 = event-data() -> ("ModuleID"=w430:i32, "Data"=w429:variant)  [unwired: 1 in]
        n182 = case shown="True" TRUE {
          tunnel: w431 -> [w432 w434]
          tunnel: w430 -> [_ w443]
          tunnel: w429 -> [_ w441]
          tunnel: [_ w438] -> w428
          tunnel: [w432 w434] -> w426
          frame False {
          }
          frame True {
            # "Find Bus Index"
            n183 = for {
              tunnel: w434 -> [w448] mode=indexing
              tunnel: w443 -> [w446]
              tunnel: [w444] -> w442
              i -> [w444]
              stop <- w445 stop-if-true
              n184 = property class="Bus.lvclass"(reference=w448) -> ("Accessors:EventModuleID"=w447:i32)  [unwired: 1 in, 2 out]
              n185 = Equal?(x=w447, y=w446) -> (x = y?=w445:bool)
            }
            n186 = Variant To Data(type=T8 [] ("ui32FlagImpairmentArray"), Variant=w441) -> (data=w439:T8)  [unwired: 1 in, 1 out]
            n187 = Bundle By Name(cluster=T20 {"BusIndex"=0, "FlagImpairArray"=[]} ("clEvtReportArray"), "BusIndex"=w442, "FlagImpairArray"=w439) -> (w437:T20)
            n188 = local read "QueName"() -> (w433:string)
            n189 = call "Enqueue.vi"("QueName"=w433, "Data"=w437, "Message"="FlagImpair") -> ("Error"=w438:errorcluster[])  [unwired: 8 in]
          }
        }
      }
      event "Scrollbar": Value Change {
        n190 = event-data() -> ("NewVal"=w450:i32)  [unwired: 1 in]
        n191 = Subtract() -> (x=w454:dbl, y=w453:dbl, x-y=w452:dbl)
        n192 = Subtract(x=w450, y=w452) -> (x-y=w451:dbl)
      }
      event "btnStop": Value Change {
        n193 = event-data() -> ()  [unwired: 1 in, 1 out]
        n194 = call "ObtainRequestEvents.vi"() -> ("Error"=w465:errorcluster[], "clRequestEvents"=w462:T9)  [unwired: 10 in]
        n195 = Unbundle By Name(w462) -> ("StopRequest"=w463:refnum<user-event>)
        n196 = Generate User Event(priority (normal)=usereventprio."high priority", user event=w463, event data cluster=T22 {"BusIndex"=0, "Data"=variant} ("event data")) -> (error out=w464:errorcluster)  [unwired: 1 in, 1 out]
        n197 = call <userlib>:"AddError.vi"("Severity"="Fatal" ("String"), "Priority"=u8 0, "ErrorArray"=w465, "error in (no error)"=w464) -> ("ErrorArray"=w461:errorcluster[], "error out"=w458:errorcluster)  [unwired: 6 in]
        n198 = call <vilib>:"Clear Errors.vi"("error in (no error)"=w458) -> ()  [unwired: 5 in, 2 out]
      }
    }
    n199 = local read "QueName"() -> (w235:string)
    n200 = call "EnqueError.vi"("QueName"=w235, "Error"=w240) -> ("Error"=w239:errorcluster[])  [unwired: 9 in]
  }
  n201 = Build Array(w28, w29) -> (→"appended array":errorcluster[][])
